vi "FF_AnkleTraj.vi"(6 "Init":bool, 8 "error in (no error)":errorcluster, 9 "AnkleVelocity":dbl[](array[numeric]), 10 "AnkleInGCS":dbl[](array[numeric]), 11 "Force Field Controller in":refnum<class "ForceField.lvclass">) -> (0 "error out":errorcluster, 1 "ClosePt":dbl[](array[numeric]), 2 "Force":dbl[](array[numeric]), 3 "Force Field Controller out":refnum<class "ForceField.lvclass">, 4 "ActiveTraj":dbl[][](array[numeric]), 5 "ForceComp":dbl[](array[numeric]))   [LabVIEW 2016, in "ForceField.lvclass"]
uses:
  ForceField.lvclass
  ForceField.lvclass/ForceField.ctl
  TypeDef/TND.ctl
panel:
  in  "HalfWindow":i32=120
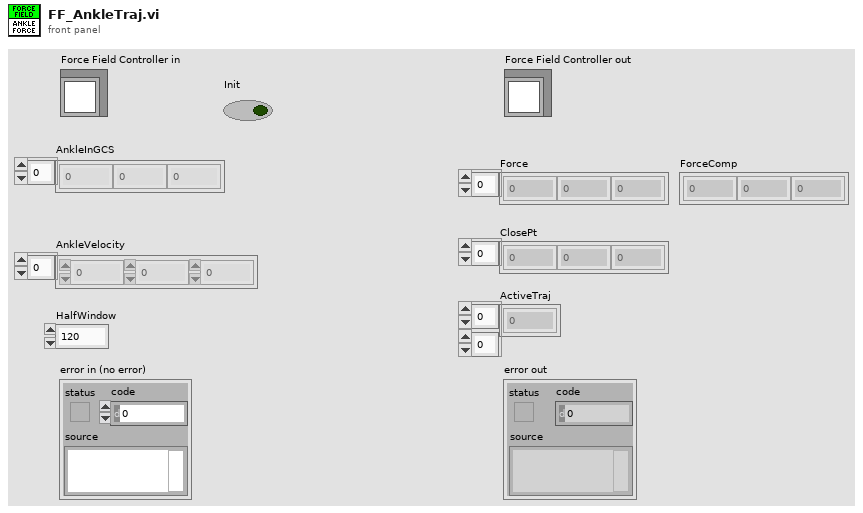
[diagram p1: front panel]
types:
  T1 = typedef "ForceField.lvclass/TND.ctl" = cluster{"Vt":dbl[], "Vn":dbl[], "Dmin":dbl}
  T2 = typedef "ForceField.lvclass/AnkleTrajPt.ctl" = cluster{"P1":dbl[], "P2":dbl[], "P1-P2":dbl[], "(P1-P2)^2":dbl}
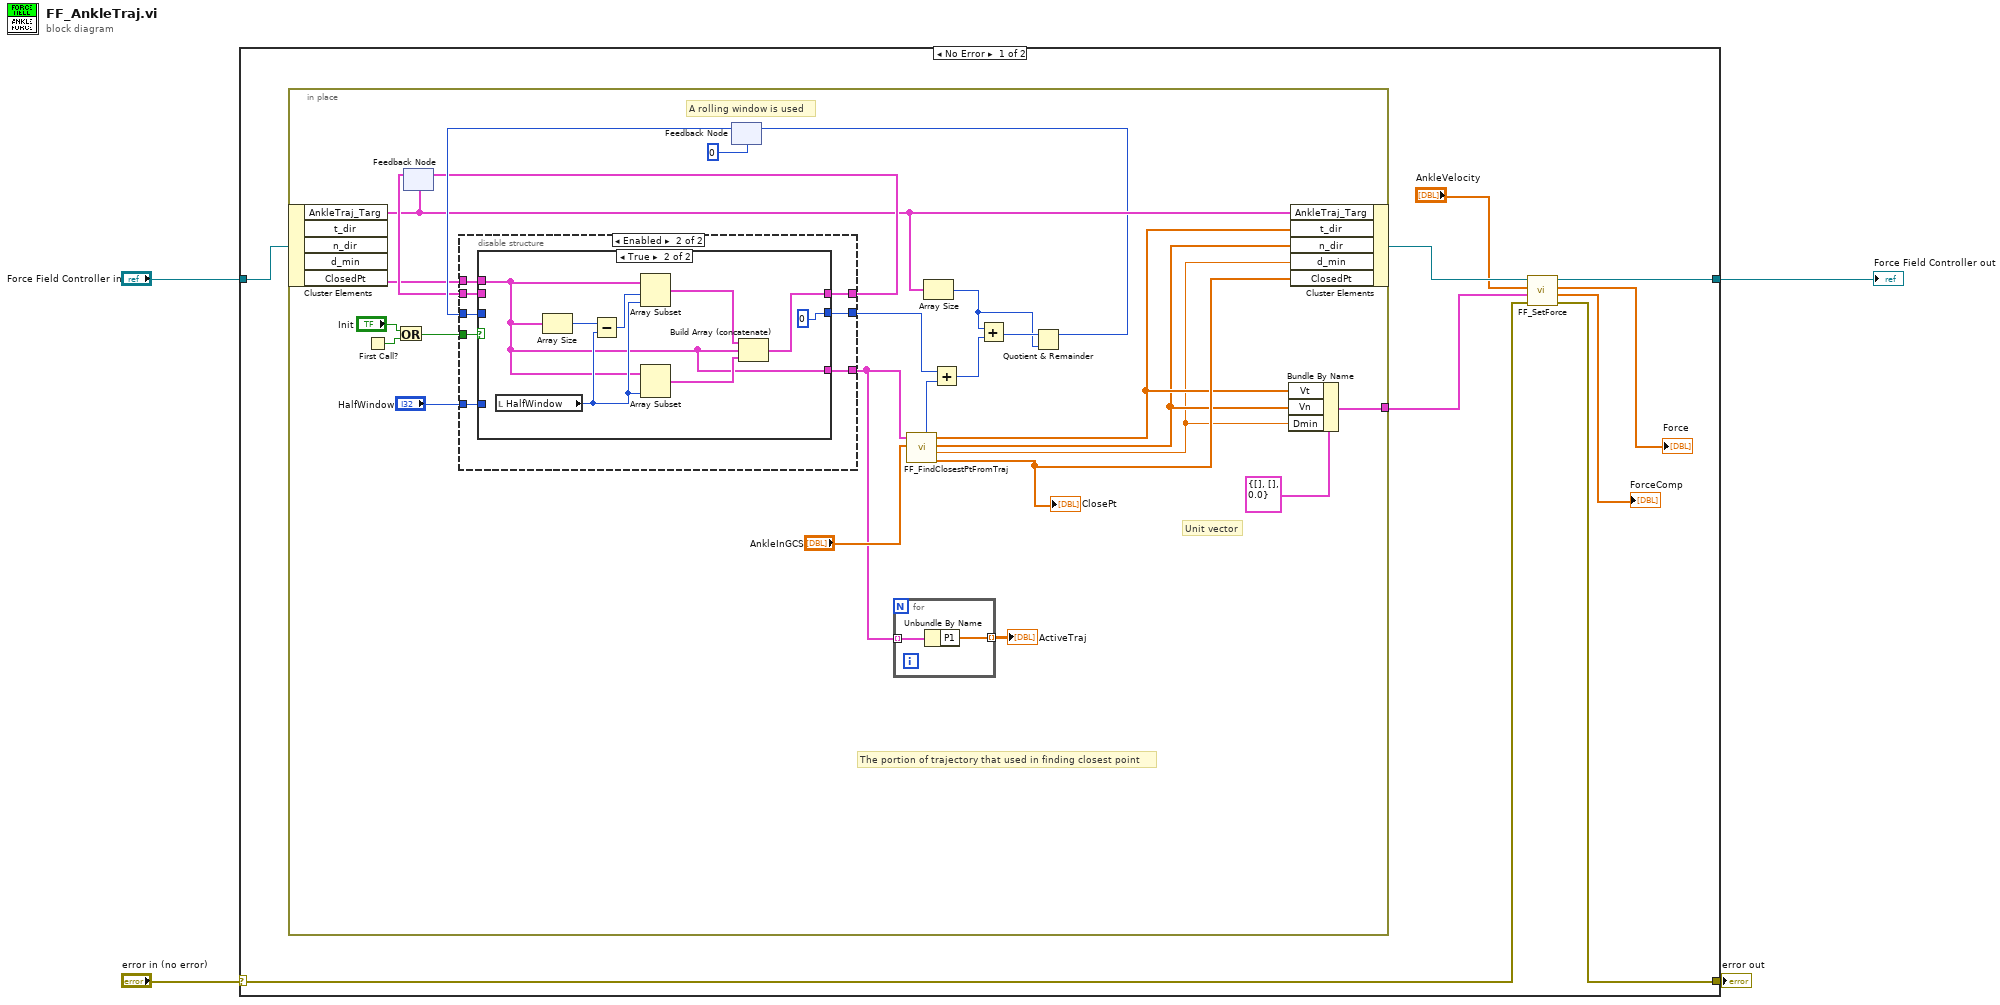
[diagram p0: block diagram]
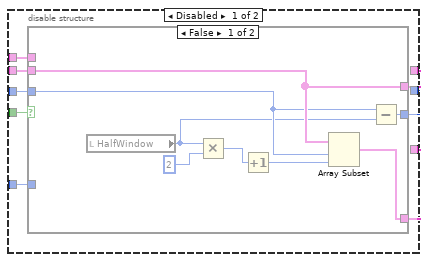
[diagram p2: hidden frame]
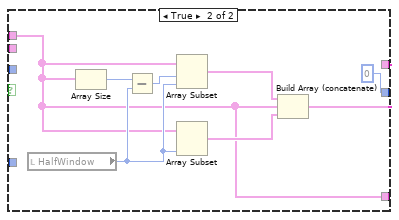
[diagram p3: hidden frame]
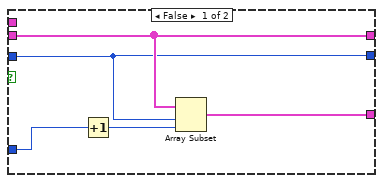
[diagram p4: hidden frame]
diagram:
  n1 = case shown="No Error" "error in (no error)" {
    selector: "error in (no error)" -> [w9 w86]
    tunnel: [w8 w86] -> w3
    tunnel: [w11 w85] -> w1
    tunnel: "Force Field Controller in" -> [w13 w85]
    frame No Error {
      n2 = in-place {
        in-place-border: [w14] -> w5
        # "A rolling window is used"
        # "The portion of trajectory that used in finding closest point"
        # "Unit vector"
        n3 = in-place-cluster #1(w13) -> ("AnkleTraj_Targ"=w31:T2[])  [unwired: 4 out]
        n4 = First Call?() -> (First Call?: T/F=w29:bool)
        n5 = Or(x="Init", y=w29) -> (x .or. y?=w27:bool)
        n6 = feedback #2(w31) -> (w34:T2[])
        n7 = feedback #3(0) -> (w36:i32)
        n8 = disable-structure shown="Enabled" {
          disable-tunnel: w27 -> [w47 w71]
          disable-tunnel: w36 -> [w46 w70]
          disable-tunnel: [w45 w69] -> w24
          disable-tunnel: w34 -> [w44 w68]
          disable-tunnel: [w43 w67] -> w33
          disable-tunnel: [w42 w66] -> w32
          disable-tunnel: w31 -> [w41 w65]
          disable-tunnel: "HalfWindow" -> [w40 w64]
          frame Disabled {
            n9 = case shown="False" w47 {
              tunnel: w46 -> [w50 _]
              tunnel: w44 -> [w54 _]
              tunnel: [w55 w56] -> w45
              tunnel: [w54 w58] -> w43
              tunnel: [w49 0] -> w42
              tunnel: w41 -> [_ w56]
              tunnel: w40 -> [_ _]
              frame False {
                n10 = local read "HalfWindow"() -> (w48:i32)
                n11 = Multiply(x=w48, y=2) -> (x*y=w53:i32)
                n12 = Increment(x=w53) -> (x+1=w52:i32)
                n13 = Array Subset(array=w54, index=w50, length=w52) -> (w55:T2[])
                n14 = Subtract(x=w50, y=w48) -> (x-y=w49:i32)
              }
              frame True {
                n15 = local read "HalfWindow"() -> (w62:i32)
                n16 = Array Size(array=w56) -> (size(s)=w63:i32)
                n17 = Subtract(x=w63, y=w62) -> (x-y=w61:i32)
                n18 = Array Subset(array=w56, index=w61, length=w62) -> (w59:T2[])
                n19 = Array Subset(array=w56, length=w62) -> (w60:T2[])  [unwired: 1 in]
                n20 = Build Array (concatenate)(w59, w56, w60) -> (w58:T2[])
              }
            }
          }
          frame Enabled {
            n21 = case shown="True" w71 {
              tunnel: w70 -> [w72 _]
              tunnel: w68 -> [w75 _]
              tunnel: [w76 w77] -> w69
              tunnel: [w75 w79] -> w67
              tunnel: [w72 0] -> w66
              tunnel: w65 -> [_ w77]
              tunnel: w64 -> [w73 _]
              frame False {
                n22 = Increment(x=w73) -> (x+1=w74:i32)
                n23 = Array Subset(array=w75, index=w72, length=w74) -> (w76:T2[])
              }
              frame True {
                n24 = local read "HalfWindow"() -> (w83:i32)
                n25 = Array Size(array=w77) -> (size(s)=w84:i32)
                n26 = Subtract(x=w84, y=w83) -> (x-y=w82:i32)
                n27 = Array Subset(array=w77, index=w82, length=w83) -> (w80:T2[])
                n28 = Array Subset(array=w77, length=w83) -> (w81:T2[])  [unwired: 1 in]
                n29 = Build Array (concatenate)(w80, w77, w81) -> (w79:T2[])
              }
            }
          }
        }
        n30 = feedback-in #2(w33) -> ()
        n31 = for {
          tunnel: w24 -> [w39] mode=indexing
          tunnel: [w38] -> w23 mode=indexing
          n32 = Unbundle By Name(w39) -> ("P1"=w38:dbl[])
        }
        "ActiveTraj" <- w23
        n33 = call "FF_FindClosestPtFromTraj.vi"("AnkleInGCS"="AnkleInGCS", "AnkleTraj"=w24) -> ("ClosestPt"=w26:dbl[], "DistanceToClosestPt"=w15:dbl, "NormalVectorToClosestPt"=w16:dbl[], "TangentVectorAtClosestPt"=w17:dbl[], "IndexOfClosePt"=w25:i32)  [unwired: 5 in]
        "ClosePt" <- w26
        n34 = Array Size(array=w31) -> (size(s)=w20:i32)
        n35 = Add(x=w32, y=w25) -> (x+y=w22:i32)
        n36 = Add(x=w20, y=w22) -> (x+y=w21:i32)
        n37 = Quotient & Remainder(x=w21, y=w20) -> (x-y*floor(x/y)=w19:i32)  [unwired: 1 out]
        n38 = feedback-in #3(w19) -> ()
        n39 = Bundle By Name(cluster=T1 {"Vt"=[], "Vn"=[], "Dmin"=0.0} ("TND"), "Vt"=w17, "Vn"=w16, "Dmin"=w15) -> (w14:T1)
        n40 = in-place-cluster #1("AnkleTraj_Targ"=w31, "t_dir"=w17, "n_dir"=w16, "d_min"=w15, "ClosedPt"=w26) -> (w12:refnum<class "ForceField.lvclass">)
      }
      n41 = call "FF_SetForce.vi"("error in (no error)"=w9, "TND"=w5, "AnkleVelocity"="AnkleVelocity", "Force Field Controller in"=w12) -> ("error out"=w8:errorcluster, "ForceNTD"=→"ForceComp":dbl[], "ForceXYZ"=→"Force":dbl[], "Force Field Controller out"=w11:refnum<class "ForceField.lvclass">)  [unwired: 4 in]
    }
    frame Error {
    }
  }
  "error out" <- w3
  "Force Field Controller out" <- w1
